vi "SystemLink Comm.vi"() -> ()   [LabVIEW 2016]
uses:
  VIs/SystemLink/ReadTagValue.vi
  VIs/SystemLink/Systemlink Tag.xctl
panel:
  in  "Systemlink Tag":T1(xcontrol)
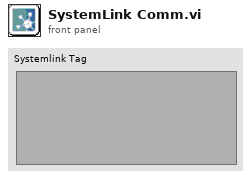
[diagram p1: front panel]
types:
  T1 = cluster{"Tag Name":string, "Type":string, "Data":string}
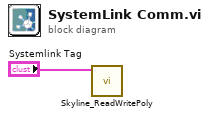
[diagram p0: block diagram]
diagram:
  n1 = call-poly "Skyline_ReadWritePoly.vi"("Tag"="Systemlink Tag") -> ()  [unwired: 9 in, 2 out]
